vi "startSweep.vi"(8 "error in (no error)":errorcluster, 11 "Instrument.Lockin in":refnum<class "Instrument.Lockin.lvclass">) -> (0 "error out":errorcluster, 3 "Instrument.Lockin out":refnum<class "Instrument.Lockin.lvclass">)   [LabVIEW 2016, in "Instrument.Lockin.lvclass"]
doc: "API to assert the trigger.\n\nIf address=\"\", this API reads from localhost\nIf address is remote lockin, you need to add this computer to allowed whitelist on the lockin computer you are trying to access."
uses:
  Instrument.Lockin.lvclass
  Instrument.Lockinl.UI/Typedefs/Lockin.Commands--Enum.ctl
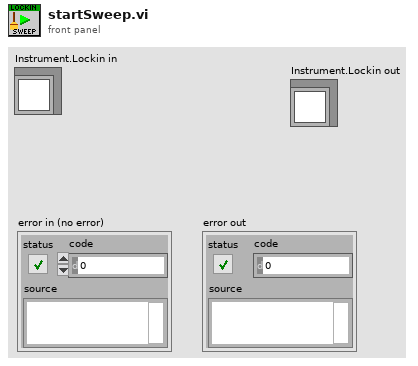
[diagram p1: front panel]
types:
  T1 = typedef "Instrument.Lockin.lvclass/Lockin.Commands--Enum.ctl" = enum16{"setAO", "setAO_Amplitude", "setAO_DC", "setAO_Frequency", "setAO_Phase", "setAO_Function", "setAO_I+", "setREF", "setREF_Frequency", "setREF_Phase", "setIVmode", "Reset", "setSampling", "Trigger", "getAO", "getAI", "getResults", "getTrigger", "getIVmode", "getSampling", "getAOconfig", "getREFconfig", "setGain", "getGain", "setAutoSampling", "getAutoSampling", "setSweep", "getStatus", "getSweepResults", "getIVSweepResults", "startSweep", "stopSweep", "setAUX", "getAUX"}
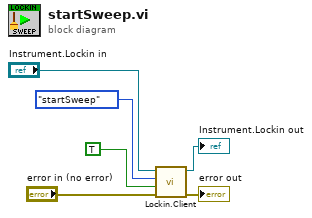
[diagram p0: block diagram]
diagram:
  n1 = call "Lockin.Client.vi"("error in (no error)"="error in (no error)", "Data"=TRUE, "Command"=Lockin.Commands--Enum."startSweep", "Instrument.Lockin in"="Instrument.Lockin in") -> ("error out"=→"error out":errorcluster, "Instrument.Lockin out"=→"Instrument.Lockin out":refnum<class "Instrument.Lockin.lvclass">)  [unwired: 5 in, 1 out]
